vi "Mouse Down V2.vi"(4 "Ground Station Operations Queue Ref":refnum<queue>, 5 "Event Data":cluster{"sender":refnum<k24>, "e":refnum<k24>}, 6 "Control Ref":refnum<k24>, 7 "Event Common Data":T1) -> ()   [LabVIEW 2014]
uses:
  C:/Robotic Systems/Products/AgFalcon/Software/Ground Station/Data/Mapping DLL/GMap.NET.WindowsForms.dll
  Data/Mapping DLL/GMap.NET.WindowsForms.dll
  System.Windows.Forms
  Application Support/Data Processing Queue/Controls/Data Queue.ctl
panel:
  out "Button":i32(ring) items=["None"=0, "Left"=1048576, "Right"=2097152, "Middle"=4194304, "XButton1"=8388608, "XButton2"=16777216]
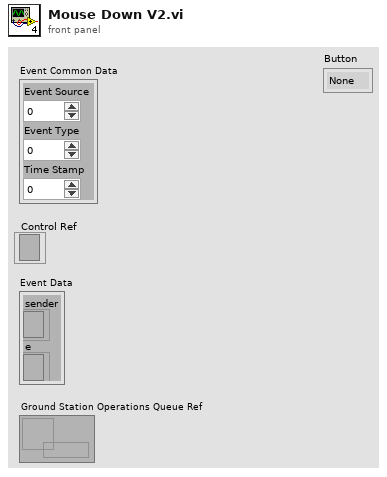
[diagram p1: front panel]
types:
  T1 = cluster{"Event Source":i32, "Event Type":u32, "Time Stamp":u32}
  T2 = typedef "Data Queue.ctl" = cluster{"Command":string, "Data":variant}
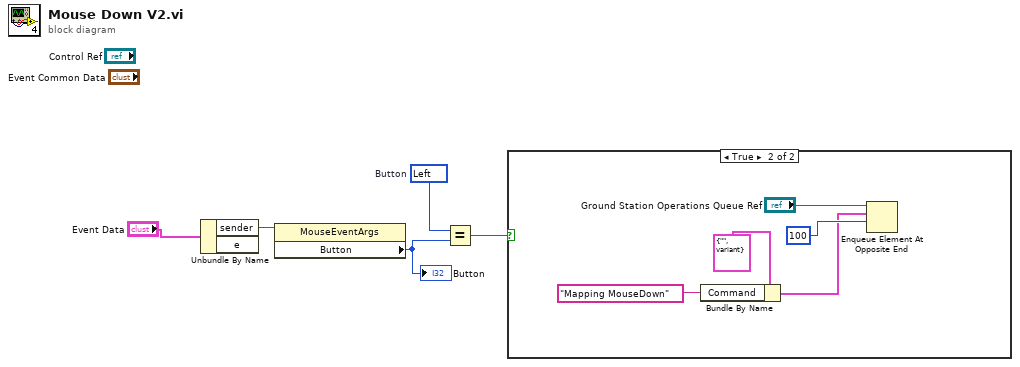
[diagram p0: block diagram]
diagram:
  w2 = 1048576 items=["None"=0, "Left"=1048576, "Right"=2097152, "Middle"=4194304, "XButton1"=8388608, "XButton2"=16777216]  # Button
  n1 = Unbundle By Name("Event Data") -> ("e"=w4:refnum<k24>)  [unwired: 1 out]
  n2 = property class="MouseEventArgs"(reference=w4) -> ("Button"=w3:i32)  [unwired: 1 in, 2 out]
  "Button" <- w3
  n3 = Equal?(x=w2, y=w3) -> (x = y?=w1:bool)
  n4 = case shown="True" w1 {
    frame False {
    }
    frame True {
      n5 = Bundle By Name(cluster=T2 {"Command"="", "Data"=variant} ("element"), "Command"="Mapping MouseDown") -> (w7:T2)
      n6 = Enqueue Element At Opposite End(queue="Ground Station Operations Queue Ref", element=w7, timeout in ms (-1)=100) -> ()  [unwired: 1 in, 3 out]
    }
  }
